vi "Write Data Type.vi"(8 "error in (no error)":errorcluster, 10 "Data Type":string, 11 "Mag Lab Result in":refnum<class "Mag Lab Result.lvclass">) -> (0 "error out":errorcluster, 3 "Mag Lab Result out":refnum<class "Mag Lab Result.lvclass">)   [LabVIEW 2015, in "Mag Lab Result.lvclass"]
uses:
  Mag Lab Result.lvclass
  Mag Lab Result.lvclass/Mag Lab Result.ctl
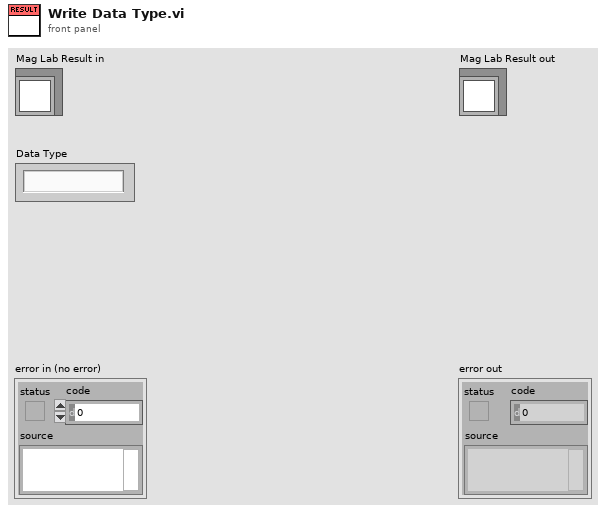
[diagram p1: front panel]
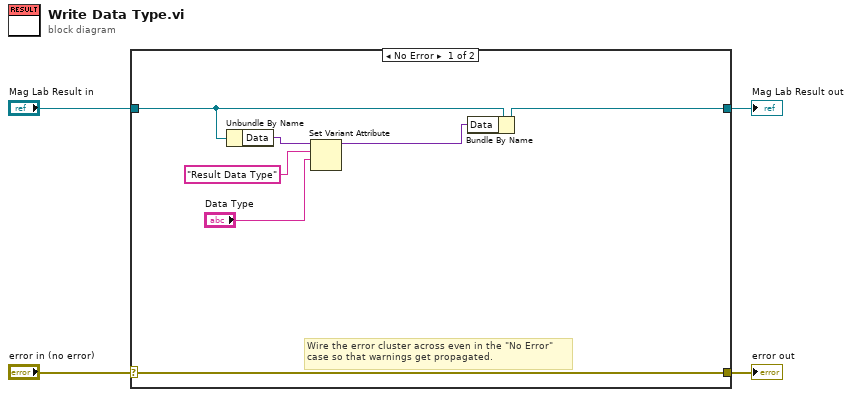
[diagram p0: block diagram]
diagram:
  n1 = case shown="No Error" "error in (no error)" {
    selector: "error in (no error)" -> [w11 w13]
    tunnel: [w11 w13] -> w3
    tunnel: [w6 w12] -> w1
    tunnel: "Mag Lab Result in" -> [w10 w12]
    frame No Error {
      # "Wire the error cluster across even in the \"No Error\"\ncase so that warnings get propagated."
      n2 = Unbundle By Name(w10) -> ("Data"=w9:variant)
      n3 = Set Variant Attribute(Variant=w9, name="Result Data Type", value="Data Type") -> (Variant out=w5:variant)  [unwired: 1 in, 2 out]
      n4 = Bundle By Name(cluster=w10, "Data"=w5) -> (w6:refnum<class "Mag Lab Result.lvclass">)
    }
    frame Error {
    }
  }
  "error out" <- w3
  "Mag Lab Result out" <- w1
